vi "ObtainSpeed.vi"(8 "error in (no error)":errorcluster, 9 "Pulses per Revolution":dbl=1.0, 10 "Counter Frequency":dbl) -> (0 "error out":errorcluster, 1 "Speed [rad/s]":dbl format="%#_10g", 2 "Speed [RPM]":dbl format="%#.6f")   [LabVIEW 2019]
panel:
  # "SubVI that allows the user to convert from a pulse frequency into a \nrotational speed (RPM or rad/s)"
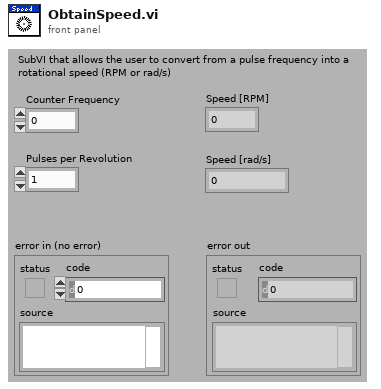
[diagram p1: front panel]
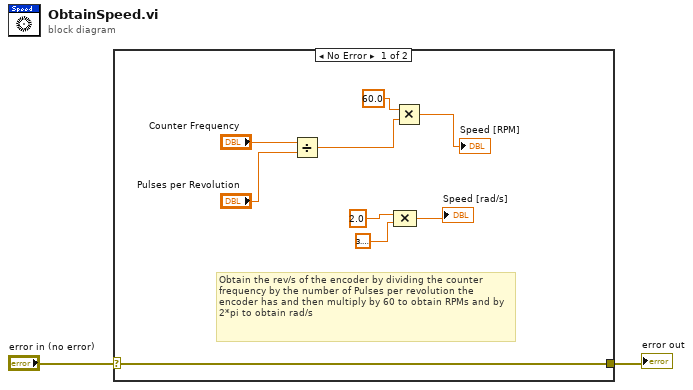
[diagram p0: block diagram]
diagram:
  n1 = case shown="No Error" "error in (no error)" {
    selector: "error in (no error)" -> [w6 w12]
    tunnel: [w6 w12] -> w1
    frame No Error {
      # "Obtain the rev/s of the encoder by dividing the counter frequency by the number of Pulses per revolution the encoder has and then multiply by 60 to obtain RPMs and by 2*pi to obtain rad/s"
      n2 = Divide(x="Counter Frequency", y="Pulses per Revolution") -> (x/y=w5:dbl)
      n3 = Multiply(x=60.0, y=w5) -> (x*y=→"Speed [RPM]":dbl)
      n4 = Compound Arithmetic op=MULTIPLY(2.0 ("value"), 3.141592653589793) -> (→"Speed [rad/s]":dbl)
    }
    frame Error {
    }
  }
  "error out" <- w1
